vi "Read Attributes.vi"(11 "Abstract Message Template in":refnum<class "Return undeliverable Msg.lvclass">) -> (2 "Payload":T2={"Tx Message"=refnum, "Tx Error"={"status"=FALSE, "code"=0, "source"=""}, "Message Priority"=enum."Normal"}, 3 "Abstract Message Template out":refnum<class "Return undeliverable Msg.lvclass">)   [LabVIEW 2014, in "Proxy.lvlib" / "Return undeliverable Msg.lvclass"]
uses:
  Return undeliverable Msg.lvclass
  <vilib>/ActorFramework/Message/Message.lvclass
  <vilib>/ActorFramework/Message Enqueuer/Message Priority.ctl
  Return undeliverable Msg.lvclass/Return undeliverable Msg.ctl
  <vilib>/ActorFramework/Message Enqueuer/Message Enqueuer.lvclass
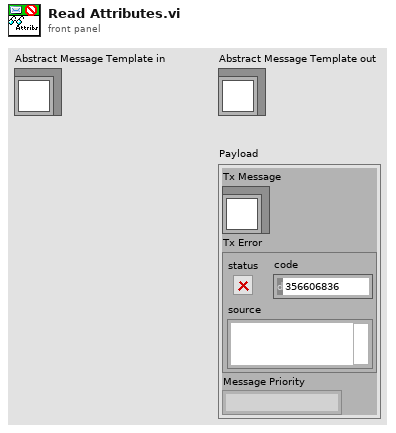
[diagram p1: front panel]
types:
  T1 = typedef "Actor Framework.lvlib/Message Enqueuer.lvclass/Message Priority.ctl" = enum16{"Low", "Normal", "High"}
  T2 = cluster{"Tx Message":refnum<class "Message.lvclass">, "Tx Error":errorcluster, "Message Priority":T1}
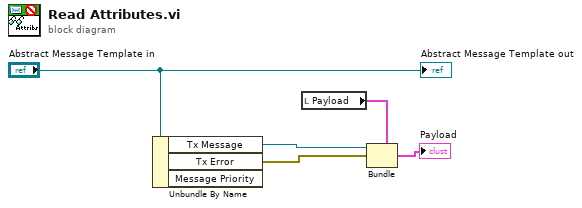
[diagram p0: block diagram]
diagram:
  n1 = Unbundle By Name("Abstract Message Template in") -> ("Tx Message"=w2:refnum<class "Message.lvclass">, "Tx Error"=w1:errorcluster)  [unwired: 1 out]
  n2 = local read "Payload"() -> (w3:T2)
  n3 = Bundle(cluster=w3, "Tx Message"=w2, "Tx Error"=w1) -> (→"Payload":T2)  [unwired: 1 in]
  "Abstract Message Template out" <- "Abstract Message Template in"
